vi "Show Main VI Core.vi"(8 "error in (no error)":errorcluster, 11 "Calling VI Ref in":refnum<vi>) -> (0 "error out":errorcluster, 3 "Calling VI Ref out":refnum<vi>)   [LabVIEW 2016]
uses:
  <vilib>/regexp/Match Regular Expression.xnode
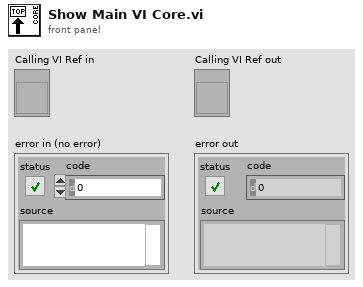
[diagram p1: front panel]
types:
  T1 = enum32{"Invalid", "Standard", "Closed", "Hidden", "Minimized", "Maximized"}
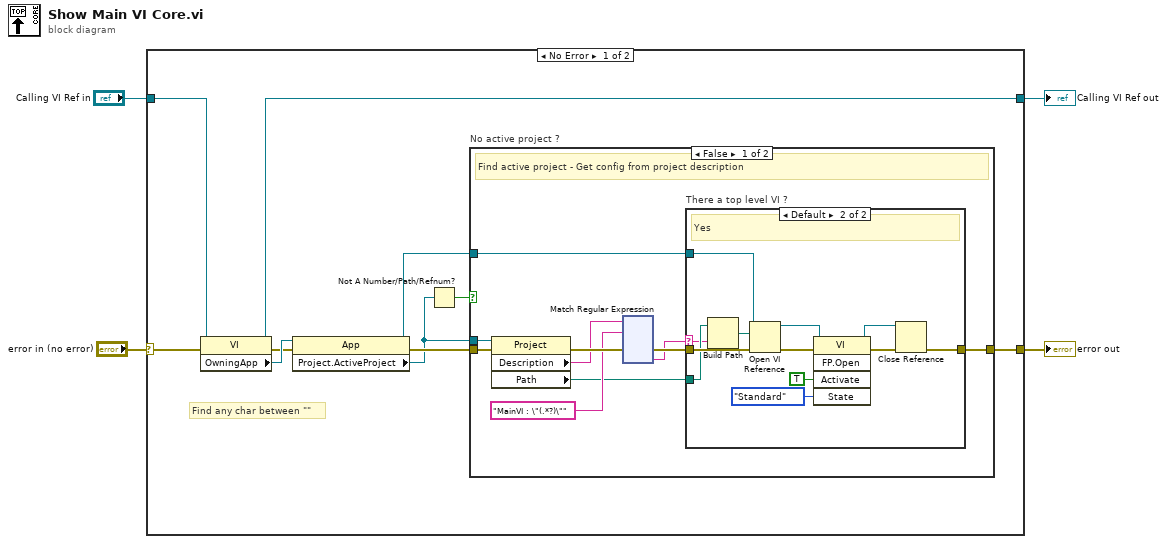
[diagram p0: block diagram]
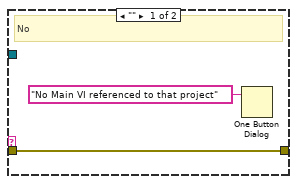
[diagram p2: hidden frame]
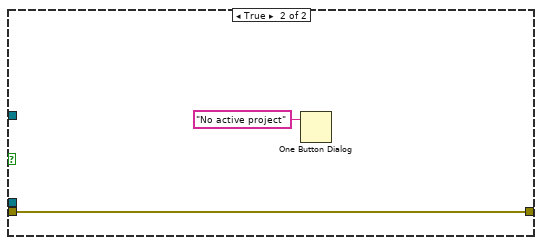
[diagram p3: hidden frame]
diagram:
  n1 = case shown="No Error" "error in (no error)" {
    selector: "error in (no error)" -> [w8 w158]
    tunnel: [w6 w158] -> w3
    tunnel: "Calling VI Ref in" -> [w7 w157]
    tunnel: [w5 w157] -> w1
    frame No Error {
      # "Find any char between \"\""
      n2 = property class="VI"(reference=w7, error in=w8) -> (reference out=w5:refnum<vi>, error out=w13:errorcluster, "OwningApp"=w14:refnum<vi>)
      n3 = property class="App"(reference=w14, error in=w13) -> (reference out=w11:refnum<vi>, error out=w12:errorcluster, "Project.ActiveProject"=w10:refnum<vi>)
      n4 = Not A Number/Path/Refnum?(number/path/refnum=w10) -> (NaN/Path/Refnum?=w9:bool)
      n5 = case "No active project ?" shown="False" w9 {
        tunnel: w12 -> [w19 w155]
        tunnel: w11 -> [w18 _]
        tunnel: [w17 w155] -> w6
        tunnel: w10 -> [w16 _]
        frame False {
          # "Find active project - Get config from project description"
          n6 = property class="Project"(reference=w16, error in=w19) -> (error out=w24:errorcluster, "Description"=w23:string, "Path"=w15:path)  [unwired: 1 out]
          n7 = xnode "Match Regular Expression"("input string"=w23, "regular expression"="MainVI : \"(.*?)\"", "error in"=w24) -> ("error out"=w21:errorcluster, "submatch 1"=w20:string)  [unwired: 3 in, 4 out]
          n8 = case "There a top level VI ?" shown="Default" w20 {
            selector: w20 -> [_ w28]
            tunnel: w21 -> [w26 w38]
            tunnel: w18 -> [_ w31]
            tunnel: [w26 w30] -> w17
            tunnel: w15 -> [_ w29]
            frame "" {
              # "No"
              n9 = One Button Dialog(message="No Main VI referenced to that project") -> ()  [unwired: 1 in, 1 out]
            }
            frame Default {
              # "Yes"
              n10 = Build Path(base path=w29, name or relative path=w28) -> (appended path=w27:path)
              n11 = Open VI Reference(application reference (local)=w31, vi path=w27, error in (no error)=w38) -> (vi reference=w35:refnum<vi>, error out=w37:errorcluster)  [unwired: 3 in]
              n12 = invoke class="VI" method="FP.Open"(reference=w35, error in=w37, "Activate"=TRUE ("Activate?"), "State"=T1."Standard") -> (reference out=w34:refnum<vi>, error out=w36:errorcluster)  [unwired: 1 in, 3 out]
              n13 = Close Reference(reference=w34, error in (no error)=w36) -> (error out=w30:errorcluster)
            }
          }
        }
        frame True {
          n14 = One Button Dialog(message="No active project") -> ()  [unwired: 1 in, 1 out]
        }
      }
    }
    frame Error {
    }
  }
  "error out" <- w3
  "Calling VI Ref out" <- w1
